vi "RT_Aerodynamic_Damping_Moment_2 (SubVI).vi"(0 "input cluster":T4, 1 "Data":dbl[][](array[numeric]), 2 "i":i32, 3 "V_wind [m/s]":dbl[][](array[numeric]), 4 "Vehicle Parameters":T2, 5 "input cluster 3":T3, 6 "Mach coeficients":dbl[](array[numeric]), 13 "Rotation":T1) -> (14 "MAd":dbl[](array[numeric]), 18 "MAd_b":dbl[](array[numeric]))   [LabVIEW 2017]
uses:
  <vilib>/Analysis/_algsub.llb/Vector Norm Type.ctl
  <vilib>/Analysis/_algsub.llb/Real Vector Norm.vi
  <vilib>/Analysis/baseanly.llb/Real A x B.vi
  <vilib>/Analysis/Matrix/Numeric/Conversions/Array To Matrix - RA2.vi
  <vilib>/Analysis/Matrix/Numeric/Conversions/Array To Matrix - RA.vi
  <vilib>/Analysis/Matrix/Numeric/Conversions/Matrix To Array - RM.vi
  <vilib>/Analysis/NI_AALPro.lvlib
  <vilib>/Analysis/NI_AALBase.lvlib
  <vilib>/Analysis/Matrix/NI_Matrix.lvlib
panel:
  out "V_norm":dbl
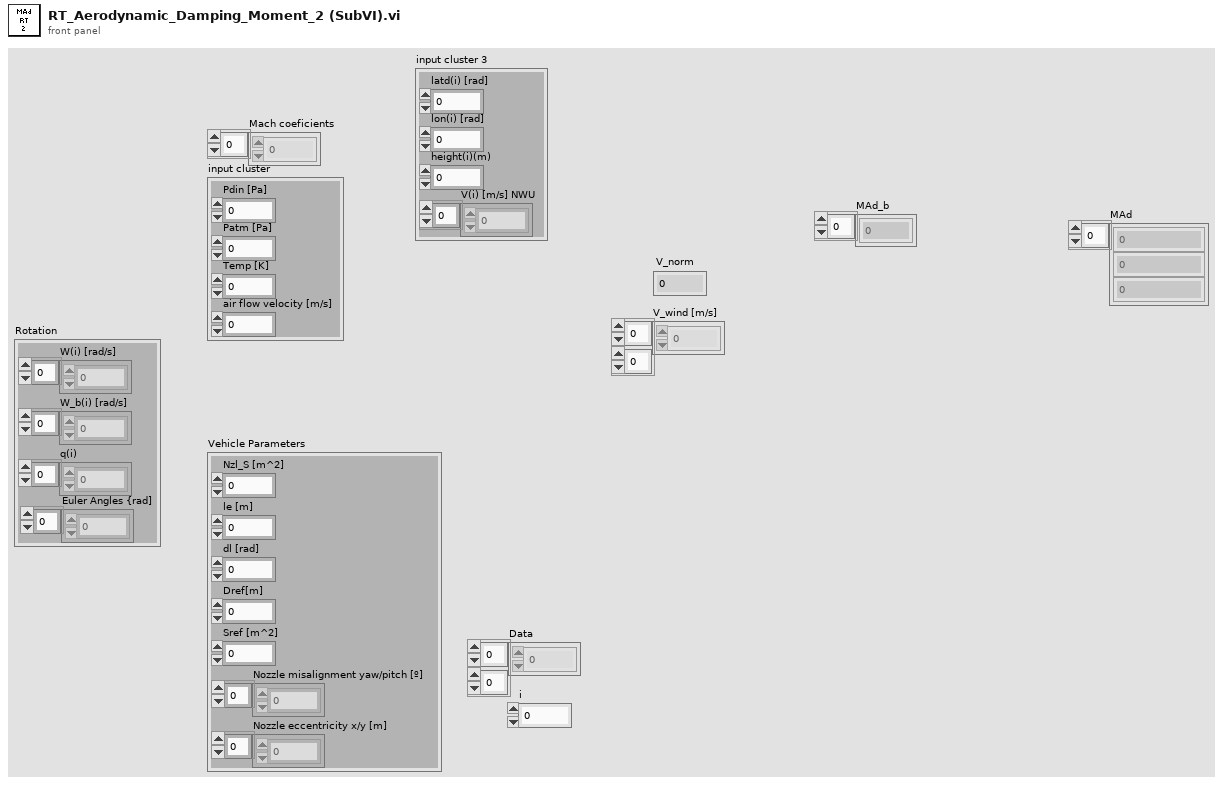
[diagram p1: front panel]
types:
  T1 = cluster{"W(i) [rad/s]":dbl[], "W_b(i) [rad/s]":dbl[], "q(i)":dbl[], "Euler Angles {rad]":dbl[]}
  T2 = cluster{"Nzl_S [m^2]":dbl, "le [m]":dbl, "dl [rad]":dbl, "Dref[m]":dbl, "Sref [m^2]":dbl, "Nozzle misalignment yaw/pitch [º]":dbl[], "Nozzle eccentricity x/y [m]":dbl[]}
  T3 = cluster{"latd(i) [rad]":dbl, "lon(i) [rad]":dbl, "height(i)(m)":dbl, "V(i) [m/s] NWU":dbl[]}
  T4 = cluster{"Pdin [Pa]":dbl, "Patm [Pa]":dbl, "Temp [K]":dbl, "air flow velocity [m/s]":dbl}
  T5 = typedef "NI_AALPro.lvlib/Vector Norm Type.ctl" = u16
  T6 = typedef "NI_Matrix.lvlib/RealMatrix.ctl" = dbl[][]
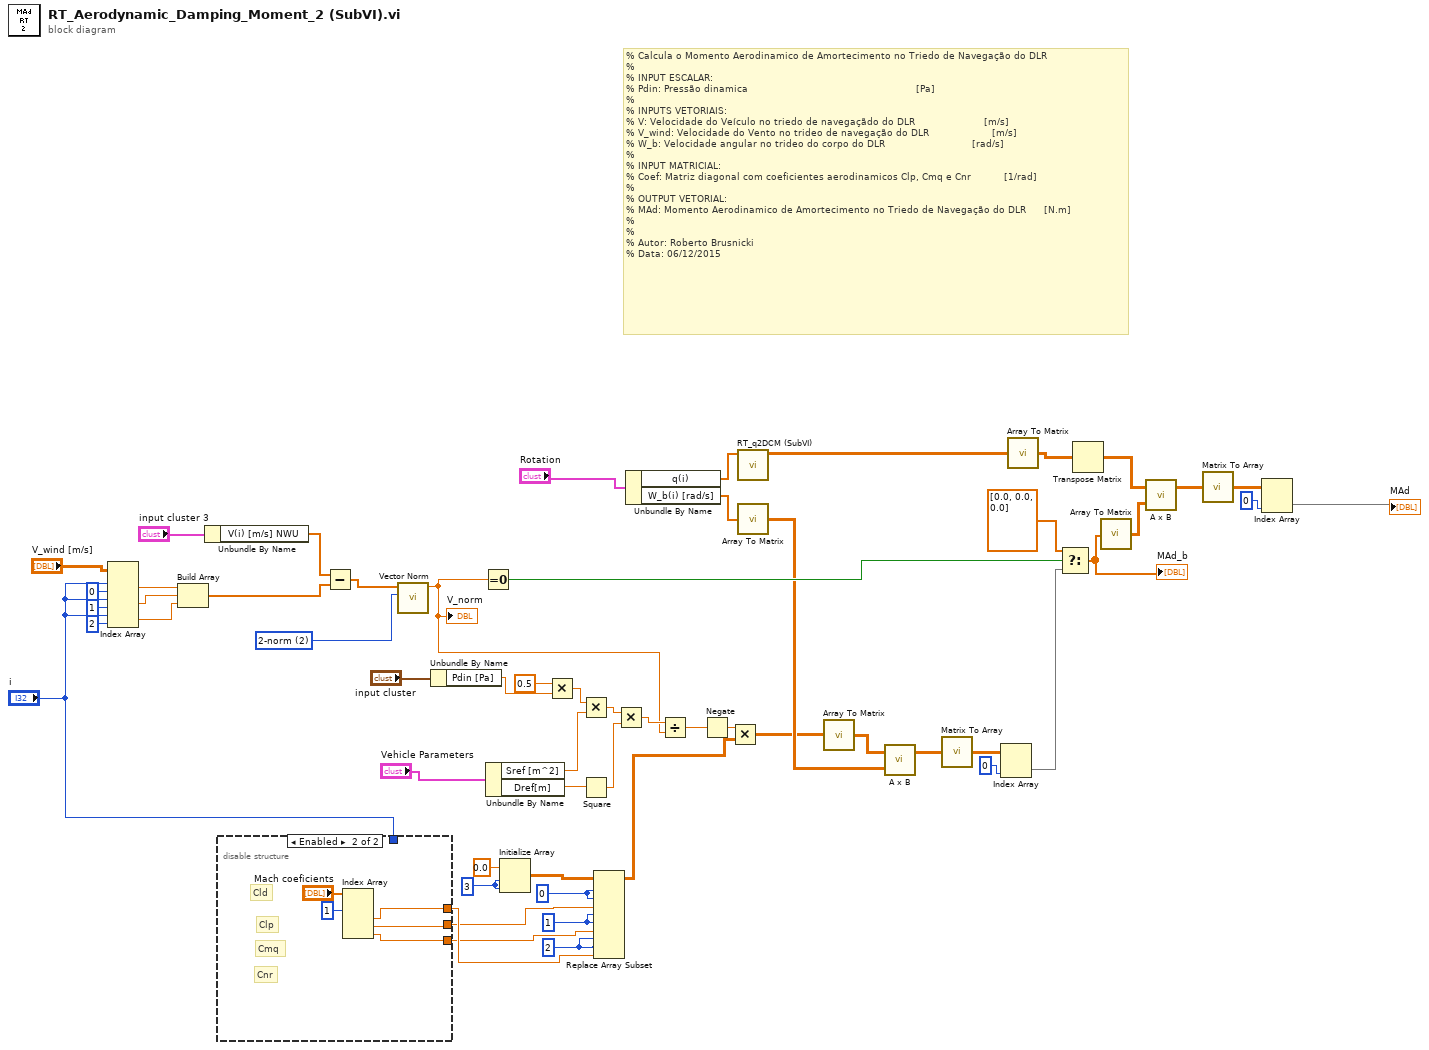
[diagram p0: block diagram]
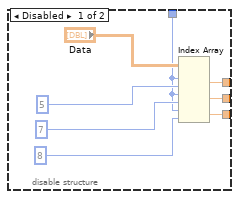
[diagram p2: hidden frame]
diagram:
  w38 = 3 ("dimension size")
  w42 = 2 ("disabled index (row)")
  w43 = 1 ("disabled index (row)")
  w41 = 0 ("disabled index (row)")
  w56 = T5 2 items=["1-norm"=1, "2-norm"=2, "Inf-norm"=3, "-Inf-norm"=4, "User Defined"=5] ("norm type")
  # "% Calcula o Momento Aerodinamico de Amortecimento no Triedo de Navegação do DLR\n%\n% INPUT ESCALAR:\n% Pdin: Pressão dinamica                                                        [Pa]\n%\n% INPUTS VETORIAIS:\n% V: Velocidade do Veículo no triedo de navegaçãdo do DLR                       [m/s]\n% V_wind: Velocidade do Vento no trideo de navegação do DLR                     [m/s]\n% W_b: Velocidade angular no trideo do corpo do DLR                             [rad/s]\n%\n% INPUT MATRICIAL:\n% Coef: Matriz diagonal com coeficientes aerodinamicos Clp, Cmq e Cnr           [1/rad]\n%\n% OUTPUT VETORIAL:\n% MAd: Momento Aerodinamico de Amortecimento no Triedo de Navegação do DLR      [N.m]\n% \n%\n% Autor: Roberto Brusnicki\n% Data: 06/12/2015"
  n1 = Index Array(array="V_wind [m/s]", index (row) #1="i", index (col) #1=0 ("disabled index (col)"), index (row) #2="i", index (col) #2=1 ("disabled index (col)"), index (row) #3="i", index (col) #3=2 ("disabled index (col)")) -> (element #1=w17:dbl, element #2=w16:dbl, element #3=w15:dbl)
  n2 = Build Array(w17, w16, w15) -> (w14:dbl[])
  n3 = Unbundle By Name("input cluster 3") -> ("V(i) [m/s] NWU"=w7:dbl[])
  n4 = disable-structure shown="Enabled" {
    disable-tunnel: [w61 w68] -> w12
    disable-tunnel: [w60 w67] -> w10
    disable-tunnel: [w59 w66] -> w11
    disable-tunnel: "i" -> [w58 _]
    frame Disabled {
      n5 = Index Array(array="Data", index (row) #1=w58, index (col) #1=5 ("disabled index (col)"), index (row) #2=w58, index (col) #2=7 ("disabled index (col)"), index (row) #3=w58, index (col) #3=8 ("disabled index (col)")) -> (element #1=w61:dbl, element #2=w60:dbl, element #3=w59:dbl)
    }
    frame Enabled {
      # "Cnr"
      # "Cmq"
      # "Clp"
      # "Cld"
      n6 = Index Array(array="Mach coeficients", index #1=1 ("index")) -> (element #2=w68:dbl, element #3=w67:dbl, element #4=w66:dbl)  [unwired: 3 in, 1 out]
    }
  }
  n7 = Subtract(x=w7, y=w14) -> (x-y=w57:dbl[])
  n8 = call-poly <vilib>:"Vector Norm.vi"("norm type"=w56, "Input Vector"=w57) -> ("norm"=w46:dbl)  [unwired: 8 in, 1 out]
  "V_norm" <- w46
  n9 = Unbundle By Name("input cluster") -> ("Pdin [Pa]"=w9:dbl)
  n10 = Equal To 0?(x=w46) -> (x = 0?=w55:bool)
  n11 = Unbundle By Name("Vehicle Parameters") -> ("Sref [m^2]"=w48:dbl, "Dref[m]"=w50:dbl)
  n12 = Initialize Array(0.0 ("element"), w38, w38) -> (w40:dbl[][])
  n13 = Multiply(x=0.5, y=w9) -> (x*y=w53:dbl)
  n14 = Multiply(x=w53, y=w48) -> (x*y=w52:dbl)
  n15 = Square(x=w50) -> (x^2=w49:dbl)
  n16 = Replace Array Subset(array=w40, new element #1=w10, index (row) #1=w41, index (col) #1=w41, new element #2=w11, index (row) #2=w43, index (col) #2=w43, new element #3=w12, index (row) #3=w42, index (col) #3=w42) -> (w37:dbl[][])
  n17 = Multiply(x=w52, y=w49) -> (x*y=w51:dbl)
  n18 = Unbundle By Name("Rotation") -> ("q(i)"=w4:dbl[], "W_b(i) [rad/s]"=w3:dbl[])
  n19 = Divide(x=w51, y=w46) -> (x/y=w45:dbl)
  n20 = Negate(x=w45) -> (-x=w44:dbl)
  n21 = Multiply(x=w44, y=w37) -> (x*y=w32:dbl[][])
  n22 = call "RT_q2DCM (SubVI).vi"("Quaternion"=w4) -> ("DCM"=w2:dbl[][])  [unwired: 10 in]
  n23 = call-poly <vilib>:"Array To Matrix.vi"("Real 1D Array"=w3) -> ("Real Matrix (Column Vector)"=w36:T6)
  n24 = call-poly <vilib>:"Array To Matrix.vi"("Real 2D Array"=w32) -> ("Real Matrix"=w31:T6)
  n25 = call-poly <vilib>:"A x B.vi"("B"=w36, "A"=w31) -> ("A x B"=w34:T6)  [unwired: 1 out]
  n26 = call-poly <vilib>:"Matrix To Array.vi"("Real Matrix"=w34) -> ("Real 2D Array"=w35:dbl[][])
  n27 = Index Array(array=w35, index (col)=0 ("index (row)")) -> (element=w30:dbl[])  [unwired: 1 in]
  n28 = call-poly <vilib>:"Array To Matrix.vi"("Real 2D Array"=w2) -> ("Real Matrix"=w24:T6)
  n29 = Select(t=dbl[] [0.0, 0.0, 0.0] ("V_wind [m/s] 2"), s=w55, f=w30) -> (s? t:f=w22:dbl[])
  "MAd_b" <- w22
  n30 = Transpose Matrix(1:w24) -> (0:w23:T6)
  n31 = call-poly <vilib>:"Array To Matrix.vi"("Real 1D Array"=w22) -> ("Real Matrix (Column Vector)"=w29:T6)
  n32 = call-poly <vilib>:"A x B.vi"("B"=w29, "A"=w23) -> ("A x B"=w27:T6)  [unwired: 1 out]
  n33 = call-poly <vilib>:"Matrix To Array.vi"("Real Matrix"=w27) -> ("Real 2D Array"=w28:dbl[][])
  n34 = Index Array(array=w28, index (col)=0 ("index (row)")) -> (element=→"MAd":dbl[])  [unwired: 1 in]
